vi "AdaptiveThreshold.vi"(4 "Kernel Block Size (Default: 5)":T1=enum."5", 5 "Adaptive Threshold Method":T2, 6 "Invert? (Default: False)":bool, 7 "Max Value (Default: 255)":u8=255, 8 "error in (no error)":errorcluster, 9 "C":dbl, 10 "Adaptive Threshold Result":refnum<data-value>, 11 "Greyscale Image-Source":refnum<data-value>) -> (0 "error out":errorcluster, 3 "Adaptive Threshold Result (duplicate)":refnum<data-value>)   [LabVIEW 2020, in "g_ar_toolkit.image.lvlib"]
uses:
  g_ar_toolkit.image.lvlib
  AdaptiveThresholdMethod.ctl
  Kernel Block Size.ctl
  g_ar_toolkit.common/g_ar_toolkit.common.lvlib
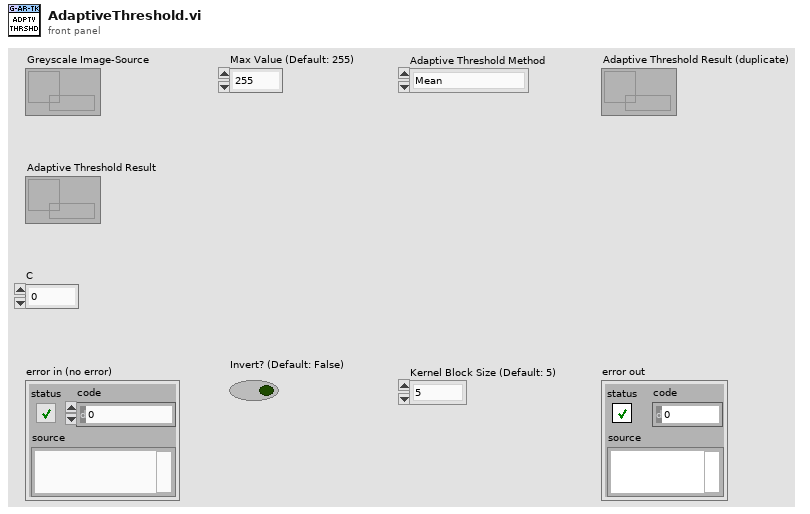
[diagram p1: front panel]
types:
  T1 = typedef "g_ar_toolkit.image.lvlib/Kernel Block Size.ctl" = enum16{"3", "5", "7", "9", "11", "13", "15", "17", "19", "21", "23", "25", "27", "29", "31", "33", "35", "37", "39", "41", "43", "45", "47", "49", "51", "53", "55", "57", "59", "61", "63", "65", "67", "69", "71", "73", "75", "77", "79", "81", "83", "85", "87", "89", "91", "93", "95", "97", "99", "101", "103", "105", "107", "109", "111", "113", "115", "117", "119", "121", "123", "125", "127", "129", "131", "133", "135", "137", "139", "141", "143", "145", "147", "149", "151", "153", "155", "157", "159", "161", "163", "165", "167", "169", "171", "173", "175", "177", "179", "181", "183", "185", "187", "189", "191", "193", "195", "197", "199", "201", "203", "205", "207", "209", "211", "213", "215", "217", "219", "221", "223", "225", "227", "229", "231", "233", "235", "237", "239", "241", "243", "245", "247", "249", "251", "253", "255", "257", "259", "261", "263", "265", "267", "269", "271", "273", "275", "277", "279", "281", "283", "285", "287", "289", "291", "293", "295", "297", "299", "301", "303", "305", "307", "309", "311", "313", "315", "317", "319", "321", "323", "325", "327", "329", "331", "333", "335", "337", "339", "341", "343", "345", "347", "349", "351", "353", "355", "357"}
  T2 = typedef "g_ar_toolkit.image.lvlib/AdaptiveThresholdMethod.ctl" = enum8{"Mean", "Gaussian"}
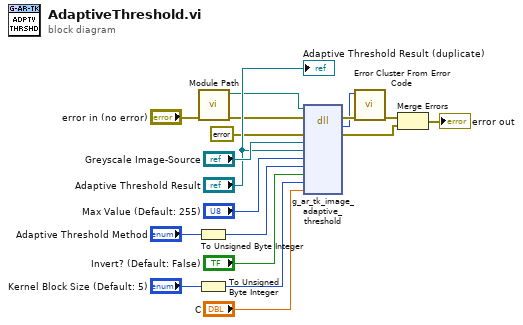
[diagram p0: block diagram]
diagram:
  n1 = To Unsigned Byte Integer(number="Adaptive Threshold Method") -> (unsigned 8bit integer=w8:u8)
  n2 = To Unsigned Byte Integer(number="Kernel Block Size (Default: 5)") -> (unsigned 8bit integer=w4:u8)
  n3 = call "Module Path.vi"("error in (no error)"="error in (no error)") -> ("error out"=w2:errorcluster, "Path"=w1:path)  [unwired: 9 in]
  n4 = dll-call lib="?" fn="g_ar_tk_image_adaptive_threshold" ("g_ar_toolkit.*.*:g_ar_tk_image_in_range")(path in=w1, error in=w2, "error_cluster"=errorcluster {"status"=FALSE, "code"=0, "source"=""} ("error constant"), "EDVR src"="Greyscale Image-Source", "EDVR dst"="Adaptive Threshold Result", "max_value"="Max Value (Default: 255)", "adaptive_method"=w8, "invert"="Invert? (Default: False)", "block_size"=w4, "c"="C") -> (error out=w14:errorcluster, "MgErr"=w13:i32, "error_cluster"=w10:errorcluster)  [unwired: 8 in, 1 out]
  n5 = call <vilib>:"Error Cluster From Error Code.vi"("error in (no error)"=w14, "error code (0)"=w13) -> ("error out"=w12:errorcluster)  [unwired: 7 in]
  n6 = Merge Errors(w12, w10) -> (→"error out":errorcluster)
  "Adaptive Threshold Result (duplicate)" <- "Adaptive Threshold Result"
